vi "WS1021 MEMS Only 24DUT Header For Design BA.vi"(8 "Error In":errorcluster) -> (0 "Error Out":errorcluster, 3 "Name Calculated Header":string[](array[string]))   [LabVIEW 2017]
panel:
  out "Measurement CS Header":string[](array[string])=["CN_Init", "B36_Cmin(fF)", "CN_1(fF)", "B36_Cmax(fF)", "CN_2(fF)", "B25_Cmin(fF)", "CN_3(fF)", "B25_Cmax(fF)", "CN_4(fF)", "12 Beams_Cmin(fF)", "CN_5(fF)", "12 Beams_Cmax(fF)", "CN_6(fF)", "ALL_Cmin(fF)", "CN_7(fF)", "ALL_Cmax(fF)", "CN_8(fF)", "B36_DeltaC(fF)", "B25_DeltaC(fF)", "12 Beams_DeltaC(fF)", "All_DeltaC(fF)", "B36_DeltaC(%)", "B25_DeltaC(%)", "12 Beams_DeltaC(%)", "All_DeltaC(%)"]
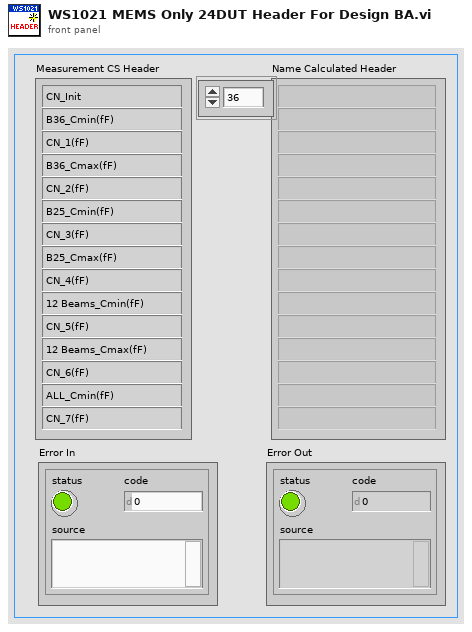
[diagram p1: front panel]
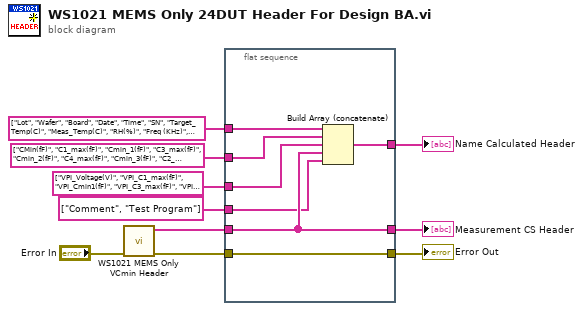
[diagram p0: block diagram]
diagram:
  n1 = call "WS1021 MEMS Only VCmin Header.vi"("Error In"="Error In") -> ("Error Out"=w4:errorcluster, "VCmin CS Header"=w3:string[])  [unwired: 9 in]
  n2 = flat-sequence {
    tunnel: w4 -> [w17]
    tunnel: [w17] -> w10
    tunnel: string[] ["Lot", "Wafer", "Board", "Date", "Time", "SN", "Target_Temp(C)", "Meas_Temp(C)", "RH(%)", "Freq (KHz)", "Stress_V(V)", "Stress_Beams", "Duty Cycle(%)", "Stress(Min/Num)"] -> [w16]
    tunnel: string[] ["CMin(fF)", "C1_max(fF)", "Cmin_1(fF)", "C3_max(fF)", "Cmin_2(fF)", "C4_max(fF)", "Cmin_3(fF)", "C2_max(fF)", "Cmin_4(fF)", "C5_max(fF)", "Cmin_5(fF)", "C6_max(fF)", "Cmin_6(fF)", "C145_max(fF)", "Cmin_7(fF)", "C236_max(fF)", "Cmin_8(fF)", "Delta_C1(fF)", "Delta_C3(fF)", "Delta_C4(fF)", "Delta_C2(fF)", "Delta_C5(fF)", "Delta_C6(fF)", "Delta_C145(fF)", "Delta_C236(fF)", "Delta_C1(%)", "Delta_C3(%)", "Delta_C4(%)", "Delta_C2(%)", "Delta_C5(%)", "Delta_C6(%)", "Delta_C145(%)", "Delta_C236(%)"] ("Measurement Header") -> [w15]
    tunnel: [w14] -> w7
    tunnel: string[] ["VPI_Voltage(V)", "VPI_C1_max(fF)", "VPI_Cmin1(fF)", "VPI_C3_max(fF)", "VPI_Cmin2(fF)", "VPI_C4_max(fF)", "VPI_Cmin3(fF)", "VPI_C2_max(fF)", "VPI_Cmin4(fF)", "VPI_C5_max(fF)", "VPI_Cmin5(fF)", "VPI_C6_max(V)", "VPI_Cmin6(fF)", "VPI_DCAP_C1(fF)", "VPI_DCAP_C3(fF)", "VPI_DCAP_C4(fF)", "VPI_DCAP_C2(fF)", "VPI_DCAP_C5(fF)", "VPI_DCAP_C6(fF)"] ("Measurement VPI Header") -> [w13]
    tunnel: w3 -> [w12]
    tunnel: [w12] -> w2
    tunnel: string[] ["Comment", "Test Program"] -> [w11]
    frame #0 {
      n3 = Build Array (concatenate)(w16, w15, w13, w12, w11) -> (w14:string[])
    }
  }
  "Name Calculated Header" <- w7
  "Error Out" <- w10
  "Measurement CS Header" <- w2
